vi "Parse Sensor Group 0.vi"(11 "stream in":u8[](array[numeric])) -> (1 "Sensor Group 0":T1 {"Infrared" format="%02x"}, 3 "stream out":u8[](array[numeric]))   [LabVIEW 2013]
doc: "Read Sensor Group 0 from a UART data stream."
uses:
  Sensor Group 0.ctl
  Bumps + Wheel Drops.ctl
  Low-Side Driver + Wheel Overcurrent.ctl
  Buttons.ctl
  Charging State.ctl
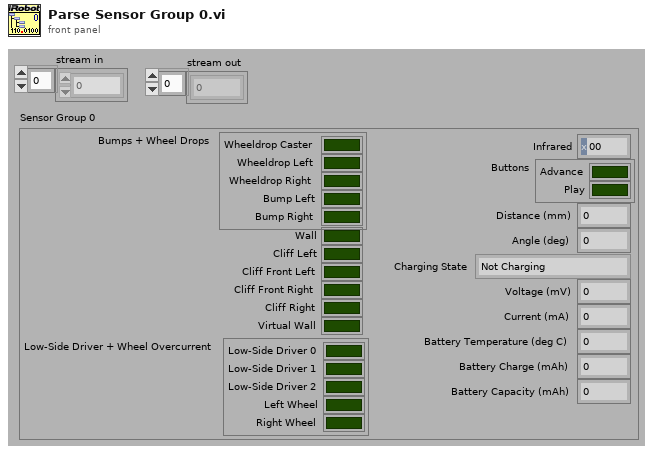
[diagram p1: front panel]
types:
  T1 = typedef "Sensor Group 0.ctl" = cluster{"Bumps + Wheel Drops":T2, "Wall":bool, "Cliff Left":bool, "Cliff Front Left":bool, "Cliff Front Right":bool, "Cliff Right":bool, "Virtual Wall":bool, "Low-Side Driver + Wheel Overcurrent":T3, "Infrared":u8, "Buttons":T4, "Distance (mm)":i32, "Angle (deg)":i32, "Charging State":T5, "Voltage (mV)":u16, "Current (mA)":i16, "Battery Temperature (deg C)":i8, "Battery Charge (mAh)":u16, "Battery Capacity (mAh)":u16}
  T2 = typedef "Bumps + Wheel Drops.ctl" = cluster{"Wheeldrop Caster":bool, "Wheeldrop Left":bool, "Wheeldrop Right":bool, "Bump Left":bool, "Bump Right":bool}
  T3 = typedef "Low-Side Driver + Wheel Overcurrent.ctl" = cluster{"Low-Side Driver 0":bool, "Low-Side Driver 1":bool, "Low-Side Driver 2":bool, "Left Wheel":bool, "Right Wheel":bool}
  T4 = typedef "Buttons.ctl" = cluster{"Advance":bool, "Play":bool}
  T5 = typedef "Charging State.ctl" = enum16{"Not Charging", "Reconditioning Charging", "Full Charging", "Trickle Charging", "Waiting", "Charging Fault Condition"}
  T6 = typedef "Sensor Group 1.ctl" = cluster{"Bumps + Wheel Drops":T2, "Wall":bool, "Cliff Left":bool, "Cliff Front Left":bool, "Cliff Front Right":bool, "Cliff Right":bool, "Virtual Wall":bool, "Low-Side Driver + Wheel Overcurrent":T3}
  T7 = typedef "Sensor Group 2.ctl" = cluster{"Infrared":u8, "Buttons":T4, "Distance (mm)":i32, "Angle (deg)":i32}
  T8 = typedef "Sensor Group 3.ctl" = cluster{"Charging State":T5, "Voltage (mV)":u16, "Current (mA)":i16, "Battery Temperature (deg C)":i8, "Battery Charge (mAh)":u16, "Battery Capacity (mAh)":u16}
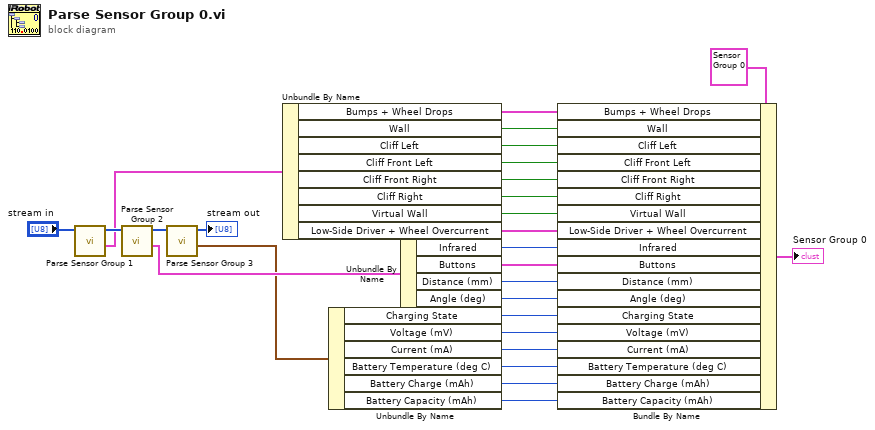
[diagram p0: block diagram]
diagram:
  n1 = call "Parse Sensor Group 1.vi"("stream in"="stream in") -> ("Sensor Group 1"=w22:T6, "stream out"=w26:u8[])  [unwired: 9 out]
  n2 = call "Parse Sensor Group 2.vi"("stream in"=w26) -> ("Sensor Group 2"=w13:T7, "stream out"=w25:u8[])  [unwired: 9 out]
  n3 = call "Parse Sensor Group 3.vi"("stream in"=w25) -> ("Sensor Group 3"=w8:T8, "stream out"=→"stream out":u8[])  [unwired: 9 out]
  n4 = Unbundle By Name(w22) -> ("Bumps + Wheel Drops"=w21:T2, "Wall"=w20:bool, "Cliff Left"=w19:bool, "Cliff Front Left"=w18:bool, "Cliff Front Right"=w17:bool, "Cliff Right"=w16:bool, "Virtual Wall"=w15:bool, "Low-Side Driver + Wheel Overcurrent"=w14:T3)
  n5 = Unbundle By Name(w8) -> ("Charging State"=w7:T5, "Voltage (mV)"=w6:u16, "Current (mA)"=w5:i16, "Battery Temperature (deg C)"=w4:i8, "Battery Charge (mAh)"=w3:u16, "Battery Capacity (mAh)"=w2:u16)
  n6 = Unbundle By Name(w13) -> ("Infrared"=w12:u8, "Buttons"=w11:T4, "Distance (mm)"=w10:i32, "Angle (deg)"=w9:i32)
  n7 = Bundle By Name(cluster=T1 {"Bumps + Wheel Drops"={"Wheeldrop Caster"=FALSE, "Wheeldrop Left"=FALSE, "Wheeldrop Right"=FALSE, "Bump Left"=FALSE, "Bump Right"=FALSE}, "Wall"=FALSE, "Cliff Left"=FALSE, "Cliff Front Left"=FALSE, "Cliff Front Right"=FALSE, "Cliff Right"=FALSE, "Virtual Wall"=FALSE, "Low-Side Driver + Wheel Overcurrent"={"Low-Side Driver 0"=FALSE, "Low-Side Driver 1"=FALSE, "Low-Side Driver 2"=FALSE, "Left Wheel"=FALSE, "Right Wheel"=FALSE}, "Infrared"=0, "Buttons"={"Advance"=FALSE, "Play"=FALSE}, "Distance (mm)"=0, "Angle (deg)"=0, "Charging State"=enum."Not Charging", "Voltage (mV)"=0, "Current (mA)"=0, "Battery Temperature (deg C)"=0, "Battery Charge (mAh)"=0, "Battery Capacity (mAh)"=0} ("Sensor Group 0"), "Bumps + Wheel Drops"=w21, "Wall"=w20, "Cliff Left"=w19, "Cliff Front Left"=w18, "Cliff Front Right"=w17, "Cliff Right"=w16, "Virtual Wall"=w15, "Low-Side Driver + Wheel Overcurrent"=w14, "Infrared"=w12, "Buttons"=w11, "Distance (mm)"=w10, "Angle (deg)"=w9, "Charging State"=w7, "Voltage (mV)"=w6, "Current (mA)"=w5, "Battery Temperature (deg C)"=w4, "Battery Charge (mAh)"=w3, "Battery Capacity (mAh)"=w2) -> (→"Sensor Group 0":T1)
